vi "Finalize.vi"(8 "error in (no error)":errorcluster, 11 "RandomNumberGenerator in":refnum<class "RandomNumberGenerator.lvclass">) -> (0 "error out":errorcluster, 3 "RandomNumberGenerator out":refnum<class "RandomNumberGenerator.lvclass">)   [LabVIEW 2020, in "RandomNumberGenerator.lvlib" / "RandomNumberGenerator.lvclass"]
doc: "<b>Finalize</b>\nThis method is called as the plugin is shut down. If there are any short-duration post-processing actions (such as writing a summary/index file of data just recorded by the plugin) or lifetime references (like DVRs of shared data used with the Handle Message method), make sure to finalize those here."
uses:
  RandomNumberGenerator.lvclass
  RandomNumberGenerator.lvclass/RandomNumberGenerator.ctl
  <vilib>/ADAS Record/Utilities/ADAS Utilities.lvlib
  C:/Program Files/National Instruments/LabVIEW 2020/vi.lib/FlexLogger/SDK/PluginSDK.lvlibp/PEFClasses/SDK/Processing Element/Processing Element.lvclass
  C:/Projects/GitHub/data-record-ad/IO Plugins/RandomNumberGenerator/PE/RandomNumberGenerator.lvclass
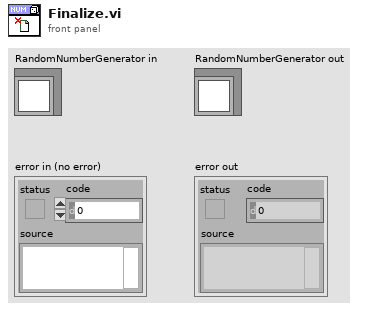
[diagram p1: front panel]
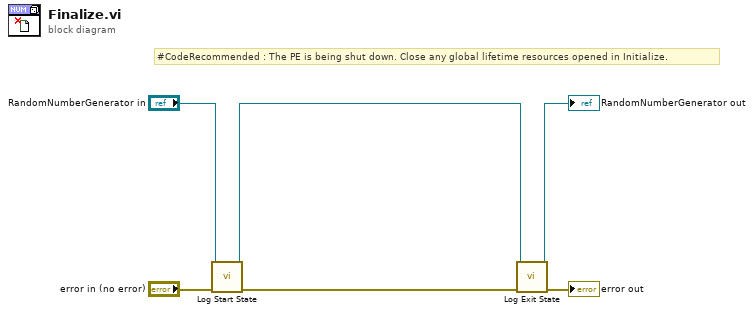
[diagram p0: block diagram]
diagram:
  # "#CodeRecommended : The PE is being shut down. Close any global lifetime resources opened in Initialize."
  n1 = call <vilib>:"Log Start State.vi"("error in (no error)"="error in (no error)", "PluginSDK.lvlibp:Processing Element.lvclass"="RandomNumberGenerator in") -> ("error out"=w5:errorcluster, "PluginSDK.lvlibp:Processing Element.lvclass"=w2:refnum<class "RandomNumberGenerator.lvclass">)  [unwired: 8 in]
  n2 = call <vilib>:"Log Exit State.vi"("error in (no error)"=w5, "PluginSDK.lvlibp:Processing Element.lvclass"=w2) -> ("error out"=→"error out":errorcluster, "PluginSDK.lvlibp:Processing Element.lvclass"=→"RandomNumberGenerator out":refnum<class "RandomNumberGenerator.lvclass">)  [unwired: 8 in]
